vi "Get message.vi"(11 "JSONMessage in":refnum<class "WampMessage JSON.lvclass">) -> (1 "<JSON>Elements":string[](array[string]), 2 "Message Type":T1, 3 "JSONMessage out":refnum<class "WampMessage JSON.lvclass">)   [LabVIEW 2020, in "wamplv.lvlib" / "WampMessage JSON.lvclass"]
uses:
  WampMessage JSON.lvclass
  TypeDefs/WAMP Message Codes.ctl
  WampMessage JSON.lvclass/WampMessage JSON.ctl
  wamplv.lvlib
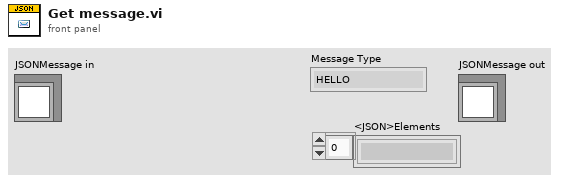
[diagram p1: front panel]
types:
  T1 = typedef "wamplv.lvlib/WAMP Message Codes.ctl" = enum8{"HELLO", "WELCOME", "CHALLENGE", "AUTHENTICATE", "ABORT", "GOODBYE", "ERROR", "PUBLISH", "PUBLISHED", "SUBSCRIBE", "SUBSCRIBED", "UNSUBSCRIBE", "UNSUBSCRIBED", "EVENT", "CALL", "RESULT", "REGISTER", "REGISTERED", "UNREGISTER", "UNREGISTERED", "INVOCATION", "YIELD"}
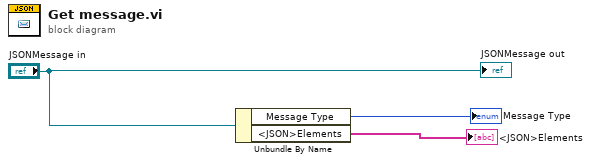
[diagram p0: block diagram]
diagram:
  n1 = Unbundle By Name("JSONMessage in") -> ("Message Type"=→"Message Type":T1, "<JSON>Elements"=→"<JSON>Elements":string[])
  "JSONMessage out" <- "JSONMessage in"
